vi "JSON to sigs 4.vi"(8 "error in":errorcluster, 11 "JSON string":string) -> (0 "error out":errorcluster, 3 "Signal Sessions":T1)   [LabVIEW 2021]
uses:
  controls/JSON sigs.ctl
  e97f2a44-d1e8-44f2-b915-a6861dd71f71.vi
  <vilib>/NI/JSON Support for LabVIEW/JSON Value/Array/Get Array Values/Get Array Values (Value[]).vi
  <vilib>/NI/JSON Support for LabVIEW/JSON Value/Read Value/Read value (String).vi
panel:
  out "Array":string[](array[string])
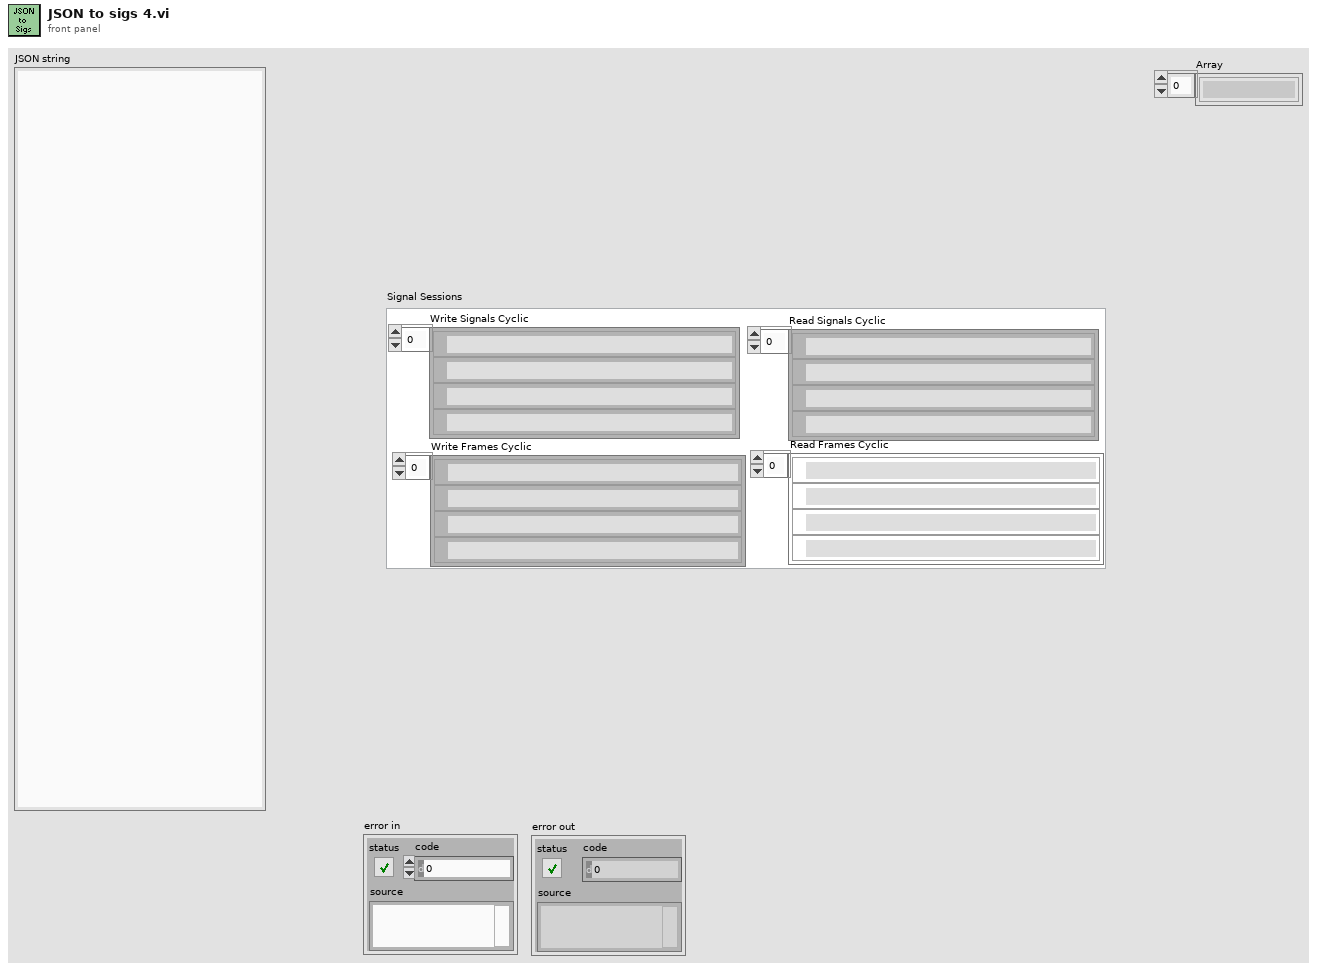
[diagram p1: front panel]
types:
  T1 = typedef "JSON sigs.ctl" = cluster{"Read Signals Cyclic":refnum<k21>[], "Write Signals Cyclic":refnum<k21>[], "Write Frames Cyclic":refnum<k21>[], "Read Frames Cyclic":refnum<k21>[]}
  T2 = cluster{"Read Signals":string, "Write Signals":string, "Init Values":string}
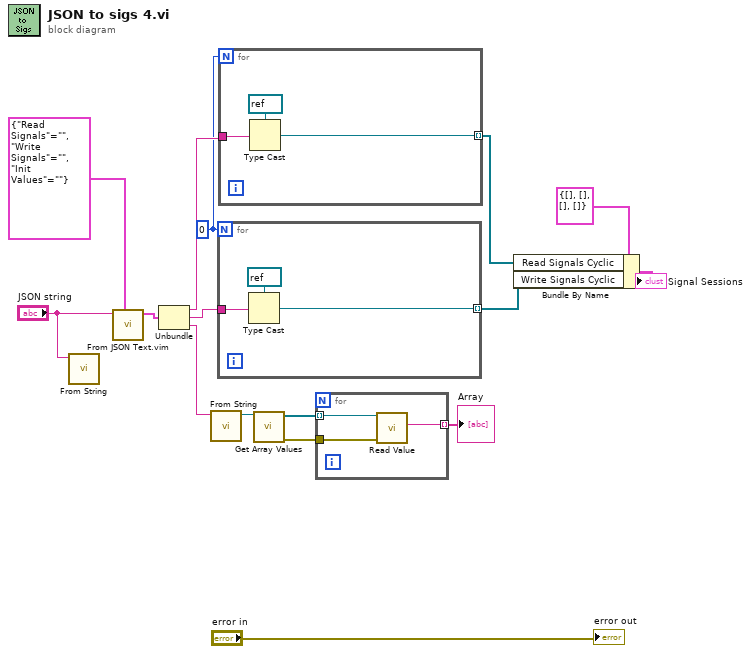
[diagram p0: block diagram]
diagram:
  w2 = 0
  n1 = call <vilib>:"From String.vi"("JSON String"="JSON string") -> ()  [unwired: 9 in, 2 out]
  n2 = call "From JSON Text.vim"("Data Type and Default Value"=T2 {"Read Signals"="", "Write Signals"="", "Init Values"=""}, "JSON"="JSON string") -> ("Data out"=w12:T2)  [unwired: 8 in, 1 out]
  n3 = Unbundle(w12) -> ("Read Signals"=w9:string, "Write Signals"=w8:string, "Init Values"=w7:string)
  n4 = call <vilib>:"From String.vi"("JSON String"=w7) -> ("JSON Value out"=w6:refnum<class "JSON Value.lvclass">)  [unwired: 9 in, 1 out]
  n5 = for {
    N: w2 -> [_]
    tunnel: w8 -> [w18]
    tunnel: [w17] -> w11 mode=indexing
    n6 = Type Cast(type=refnum<k21> refnum ("XNET Signal"), x=w18) -> (*(type *) &x=w17:refnum<k21>)
  }
  n7 = for {
    N: w2 -> [_]
    tunnel: w9 -> [w21]
    tunnel: [w20] -> w10 mode=indexing
    n8 = Type Cast(type=refnum<k21> refnum ("XNET Signal"), x=w21) -> (*(type *) &x=w20:refnum<k21>)
  }
  n9 = call-poly <vilib>:"Get Array Values.vi"("JSON Value in"=w6) -> ("error out"=w5:errorcluster, "values"=w4:refnum<class "JSON Value.lvclass">[])  [unwired: 7 in, 2 out]
  n10 = for {
    tunnel: w5 -> [w25]
    tunnel: w4 -> [w24] mode=indexing
    tunnel: [w23] -> w3 mode=indexing
    n11 = call-poly <vilib>:"Read Value.vi"("error in (no error)"=w25, "JSON String in"=w24) -> ("value"=w23:string)  [unwired: 7 in, 2 out]
  }
  "Array" <- w3
  n12 = Bundle By Name(cluster=T1 {"Read Signals Cyclic"=[], "Write Signals Cyclic"=[], "Write Frames Cyclic"=[], "Read Frames Cyclic"=[]} ("Signal Sessions"), "Read Signals Cyclic"=w10, "Write Signals Cyclic"=w11) -> (→"Signal Sessions":T1)
  "error out" <- "error in"
